vi "example.vi"() -> ()   [LabVIEW 2013]
uses:
  result/result.lvclass
  standard action/wait action/wait action.lvclass
  dispatcher/pool sizes.ctl
  dispatcher/execution system.ctl
  task/task.lvclass/task.ctl
  result/result.lvclass/result.ctl
  result/get data.vi
  result/get error.vi
  result/get generating action.vi
  result/get owning task.vi
  result/get subresults.vi
  dispatcher/thread pool.lvclass
  standard reporters/event reporter/event reporter.lvclass
  standard tasks/function task/function task.lvclass
  task/task.lvclass
panel:
  out "subresults":refnum<class "result.lvclass">[](array[class])
  out "owning task":string
  out "generating action":string
  out "error":errorcluster
  out "data":variant
  out "Time":u32
  out "result":refnum<class "result.lvclass">
  out "error out":errorcluster
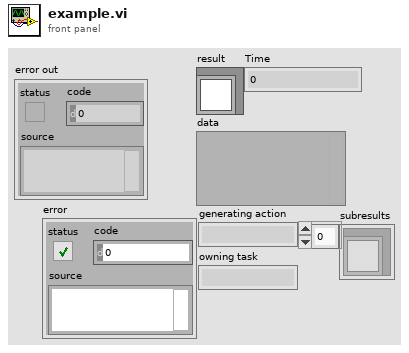
[diagram p1: front panel]
types:
  T1 = typedef "thread pool.lvclass/execution system.ctl" = enum32{"user interface", "standard", "instrument i/o", "data acquisition", "other 1", "other 2"}
  T2 = typedef "thread pool.lvclass/pool sizes.ctl" = cluster{"UI thread":u8, "standard":u8, "instrument I/O":u8, "data acquisition":u8, "other 1":u8, "other 2":u8}
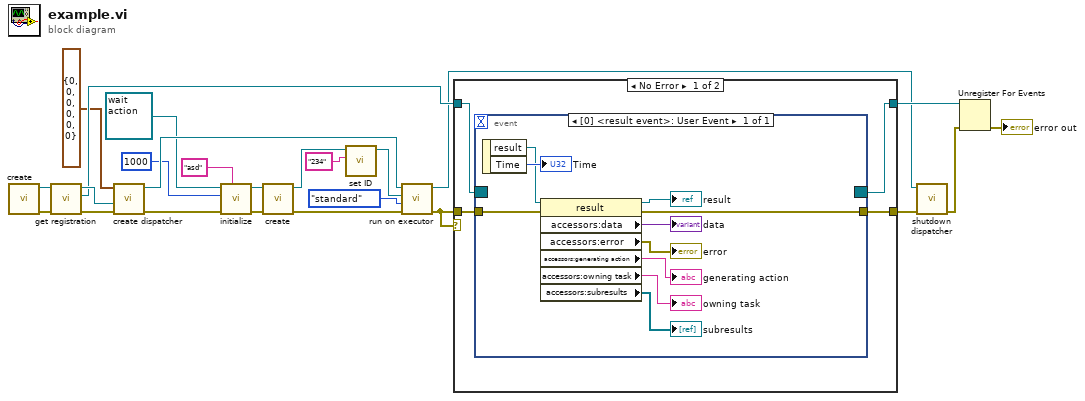
[diagram p0: block diagram]
diagram:
  n1 = call "create.vi"() -> ("error out"=w18:errorcluster, "event reporter out"=w19:refnum<class "event reporter.lvclass">)  [unwired: 10 in]
  n2 = call "get registration.vi"("error in"=w18, "event reporter in"=w19) -> ("error out"=w16:errorcluster, "result registration"=w15:refnum<event-registration>, "event reporter out"=w17:refnum<class "event reporter.lvclass">)  [unwired: 7 in]
  n3 = call "create dispatcher.vi"("error in"=w16, "default reporter"=w17, "initial pool sizes"=T2 {"UI thread"=0, "standard"=0, "instrument I/O"=0, "data acquisition"=0, "other 1"=0, "other 2"=0}) -> ("error out"=w21:errorcluster, "dispatcher"=w23:refnum<data-value>)  [unwired: 7 in]
  n4 = call-dynamic "initialize.vi"("action name"="asd", "error in"=w21, "parameters"=1000, "action in"=refnum<class "wait action.lvclass"> refnum ("wait action.lvclass")) -> ("error out"=w4:errorcluster, "action out"=w9:refnum<class "wait action.lvclass">)  [unwired: 6 in]
  n5 = call "create.vi"("action"=w9) -> ("function task out"=w8:refnum<class "function task.lvclass">)  [unwired: 10 in]
  n6 = call "set ID.vi"("ID"="234", "task in"=w8) -> ("task out"=w7:refnum<class "function task.lvclass">)  [unwired: 9 in]
  n7 = call "run on executor.vi"("error in"=w4, "execution system"=execution_system."standard", "task"=w7, "dispatcher"=w23) -> ("error out"=w3:errorcluster, "dispatcher out"=w13:refnum<data-value>)  [unwired: 6 in]
  n8 = case shown="No Error" w3 {
    tunnel: w15 -> [w27 w39]
    tunnel: [w26 w39] -> w14
    tunnel: [w25 w38] -> w10
    tunnel: w3 -> [w24 w38]
    frame No Error {
      n9 = event shown="[0] <result event>: User Event" {
        selector: w27 -> [_]
        dyn-events: [_] -> w26
        timeout: _ -> [_]
        tunnel: [w35] -> w25
        tunnel: w24 -> [w36]
        event User Event {
          n10 = event-data() -> ("result"=w34:refnum<class "result.lvclass">, "Time"=→"Time":u32)  [unwired: 1 in]
          n11 = property class="result"(reference=w34, error in=w36) -> (reference out=→"result":refnum<class "result.lvclass">, error out=w35:errorcluster, "accessors:data"=→"data":variant, "accessors:error"=→"error":errorcluster, "accessors:generating action"=→"generating action":string, "accessors:owning task"=→"owning task":string, "accessors:subresults"=→"subresults":refnum<class "result.lvclass">[])
        }
      }
    }
    frame Error {
    }
  }
  n12 = call "shutdown dispatcher.vi"("error in"=w10, "dispatcher"=w13) -> ("error out"=w12:errorcluster)  [unwired: 9 in]
  n13 = Unregister For Events(event registration refnum=w14, error in=w12) -> (error out=→"error out":errorcluster)
